vi "Apply_8V_to_J5001-T5002.vi"(3 "error in":errorcluster) -> (10 "error out":errorcluster)   [LabVIEW 2015]
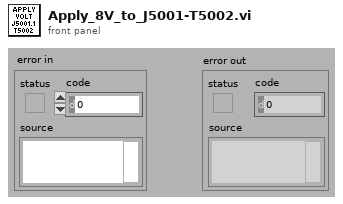
[diagram p1: front panel]
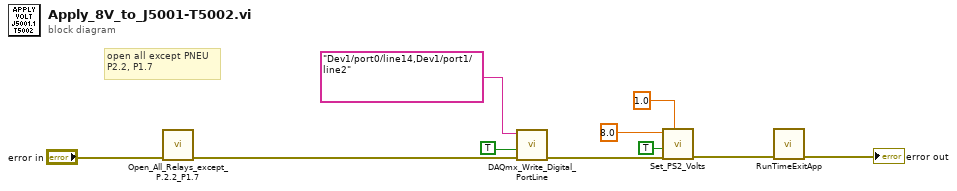
[diagram p0: block diagram]
diagram:
  # "open all except PNEU\nP2.2, P1.7"
  n1 = call "Open_All_Relays_except_P.2.2_P1.7.vi"("error in"="error in") -> ("error out"=w5:errorcluster)  [unwired: 8 in]
  n2 = call "DAQmx_Write_Digital_PortLine.vi"("Device/Ports/Lines"="Dev1/port0/line14,Dev1/port1/line2", "Boolean"=TRUE, "error in"=w5) -> ("error out"=w9:errorcluster)  [unwired: 6 in, 1 out]
  n3 = call "Set_PS2_Volts.vi"("delay (secs)"=1.0, "error in"=w9, "Output on/off"=TRUE, "Output Voltage"=8.0 ("Output Voltage (0)")) -> ("error out"=w2:errorcluster)  [unwired: 5 in, 2 out]
  n4 = call "RunTimeExitApp.vi"("error in (no error)"=w2) -> ("error out"=→"error out":errorcluster)  [unwired: 10 in]
